vi "0_Camera_Acquisition_and_Image_Saving.vi"() -> ()   [LabVIEW 2020]
doc: "Overview: This example demonstrates usage of Deep Learning Toolkit for object detection based on pretrained network called YOLO https://pjreddie.com/darknet/yolo/\nToolkit's API is utilized to automatically create network architecture based network topology configuration file and load and initialize network's weights from weight file.\nRequirements: \n1. Deep Learning Toolkit for LabVIEW\n2. NI Vision Development Module"
uses:
  subVIs/Camera/Controls/Camera_Settings.ctl
  <vilib>/vision/driver/IMAQdx.llb/IMAQdx Camera Control Mode.ctl
  <vilib>/vision/driver/NI_Vision_Acquisition_Software.lvlib
panel:
  in  "Start Index":i32
  out "Loop Time":cluster{sgl, dbl}(graph)={0.28, 0.11247559999998202}
  out "Expected Time":sgl=0.28
  in  "Table Rot. Period":sgl=5.0
  in  "Label":string="good"
  in  "Camera_Settings":T1={"Camera_Resolution"=76, "Focus"=0, "Exposure"=2, "Gain"=13, "WhiteB."=5000} {"WhiteB." min=2800 max=6500 step=1; "Gain" max=255 step=1; "Exposure" min=0 max=6 step=1; "Focus" step=17}
  in  "# Imgs to Save":i32=25
  out "Count":i32=25
  in  "Start Saving?":bool
  out "Original_Image":T2(plugin-control)
  out "Processed_Image":T2(plugin-control)
  in  "Center Crop Size":i32=900
  in  "Dest. Folder":path=path "D:/Dataset_test"
  out "Loop Time (s)":dbl=0.11247559999998202
  in  "Stop":bool
  in  "Camera":refnum<k21>="cam1" caption="IMAQdx Session"
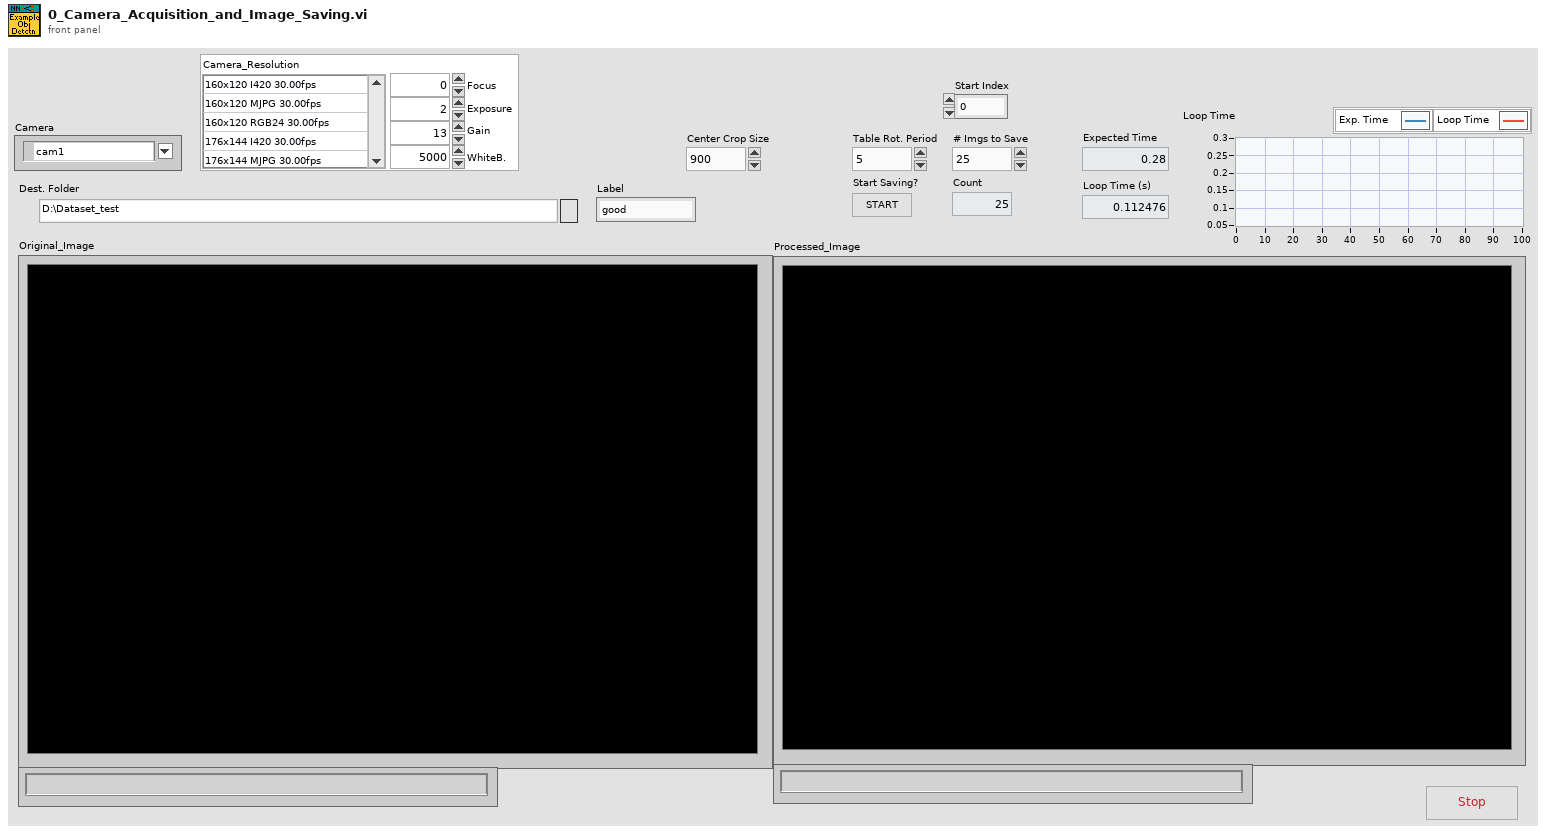
[diagram p1: front panel]
types:
  T1 = typedef "Camera_Settings.ctl" = cluster{"Camera_Resolution":i32, "Focus":u8, "Exposure":i32, "Gain":u32, "WhiteB.":i32}
  T2 = typedef "IMAQ Image.ctl" = refnum<image>
  T3 = typedef "NI_Vision_Acquisition_Software.lvlib/IMAQdx Camera Control Mode.ctl" = enum32{"Controller", "Listener"}
  T4 = typedef "Image Type" = u32
  T5 = typedef "IMAQdx.ctl" = refnum<k21>
  T6 = typedef "imagedata.ctl" = cluster{"image type":i32, "image depth":i32, "image":u8[], "mask":u8[], "colors":u32[], "Rectangle":cluster{"left":i16, "top":i16, "right":i16, "bottom":i16}}
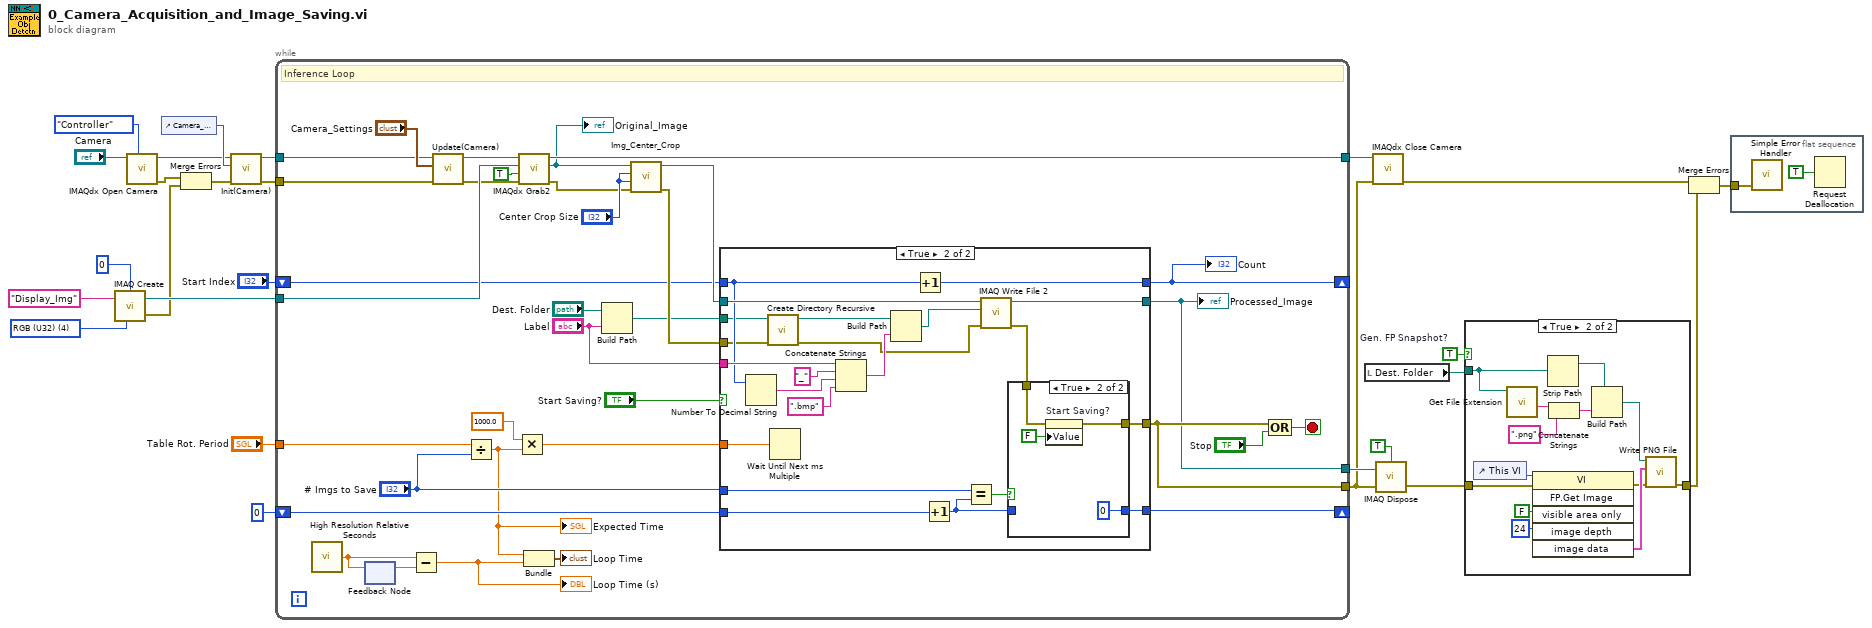
[diagram p0: block diagram]
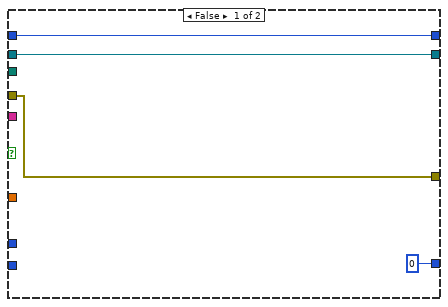
[diagram p2: hidden frame]
diagram:
  w4 = TRUE  # Gen. FP Snapshot?
  w18 = T4 4 items=["Grayscale (U8)", "Grayscale (I16)", "Grayscale (SGL)", "Complex (CSG)", "RGB (U32)", "HSL (U32)", "RGB (U64)", "Grayscale (U16)"] ("Image Type")
  n1 = call "IMAQ Create"("Border Size"=0, "Image Name"="Display_Img", "Image Type"=w18) -> ("New Image"=w24:T2, "error out"=w8:errorcluster)  [unwired: 2 in]
  n2 = call <vilib>:"IMAQdx Open Camera.vi"("Camera Control Mode"=IMAQdx_Camera_Control_Mode."Controller", "Session In"="Camera") -> ("error out"=w9:errorcluster, "Session Out"=w10:T5)  [unwired: 1 in, 7 out]
  n3 = control-ref of="Camera_Settings"() -> (w11:refnum<vi>)
  n4 = Merge Errors(w9, w8) -> (w12:errorcluster)
  n5 = call "Init(Camera).vi"("error in (no error)"=w12, "Camera_Settings_Ref"=w11, "Session in"=w10) -> ("error out"=w6:errorcluster, "Session out"=w7:T5)  [unwired: 7 in]
  n6 = while {
    tunnel: [w43] -> w25
    tunnel: w24 -> [w55]
    tunnel: [w57] -> w20
    tunnel: [w49] -> w14
    shift-right: [w48] -> _
    shift-left: "Start Index" -> [w47]
    tunnel: "Table Rot. Period" -> [w45]
    tunnel: w7 -> [w40]
    tunnel: w6 -> [w39]
    shift-right: [w31] -> _
    shift-left: 0 ("Camera Resolution") -> [w32]
    stop <- w58 stop-if-true
    # "Inference Loop"
    n7 = call <vilib>:"High Resolution Relative Seconds.vi"() -> ("relative seconds"=w59:dbl)
    n8 = feedback #1() -> (w60:dbl)  [unwired: 1 in]
    n9 = feedback-in #1(w59) -> ()
    n10 = Subtract(x=w59, y=w60) -> (x-y=w30:dbl)
    "Loop Time (s)" <- w30
    n11 = call "Update(Camera).vi"("error in (no error)"=w39, "Camera_Settings"="Camera_Settings", "Session in"=w40) -> ("error out"=w37:errorcluster, "Session out"=w38:T5)  [unwired: 7 in]
    n12 = Divide(x=w45, y="# Imgs to Save") -> (x/y=w27:sgl)
    "Expected Time" <- w27
    n13 = Multiply(x=sgl 1000.0, y=w27) -> (x*y=w28:sgl)
    n14 = call <vilib>:"IMAQdx Grab2.vi"("error in"=w37, "Wait for Next Buffer? (Yes)"=TRUE, "Image In"=w55, "Session In"=w38) -> ("error out"=w36:errorcluster, "Image Out"=w53:T2, "Session Out"=w57:T5)  [unwired: 4 in, 1 out]
    "Original_Image" <- w53
    n15 = Bundle(w27, w30) -> (→"Loop Time":cluster{sgl, dbl})  [unwired: 1 in]
    n16 = Build Path(base path="Dest. Folder", name or relative path="Label") -> (appended path=w34:path)
    n17 = call "Img_Center_Crop.vi"("error in (no error)"=w36, "height"="Center Crop Size", "width"="Center Crop Size", "Image In"=w53) -> ("error out"=w51:errorcluster, "Image Out"=w54:T2)  [unwired: 6 in]
    n18 = case shown="True" "Start Saving?" {
      tunnel: [w63 w75] -> w49
      tunnel: w34 -> [_ w68]
      tunnel: w54 -> [w64 w86]
      tunnel: [w64 w85] -> w43
      tunnel: w51 -> [w63 w66]
      tunnel: [w62 w73] -> w48
      tunnel: w47 -> [w62 w81]
      tunnel: "# Imgs to Save" -> [_ w84]
      tunnel: w28 -> [_ w83]
      tunnel: "Label" -> [_ w82]
      tunnel: w32 -> [_ w72]
      tunnel: [0 ("Camera Resolution") w71] -> w31
      frame False {
      }
      frame True {
        n19 = Number To Decimal String(number=w81) -> (decimal integer string=w80:string)  [unwired: 1 in]
        n20 = call <vilib>:"Create Directory Recursive.vi"("error in (no error)"=w66, "directory"=w68) -> ("error out"=w65:errorcluster, "directory copy"=w67:path)  [unwired: 3 in, 1 out]
        n21 = Wait Until Next ms Multiple(millisecond multiple=w83) -> ()  [unwired: 1 out]
        n22 = Concatenate Strings(w82, "_" ("string"), w80, ".bmp") -> (w78:string)
        n23 = Build Path(base path=w67, name or relative path=w78) -> (appended path=w69:path)
        n24 = Increment(x=w81) -> (x+1=w73:i32)
        n25 = Increment(x=w72) -> (x+1=w70:i32)
        n26 = Equal?(x=w84, y=w70) -> (x = y?=w77:bool)
        n27 = call-poly "IMAQ Write File 2"("error in (no error)"=w65, "File Path"=w69, "Image"=w86) -> ("error out"=w76:errorcluster, "Image Out (duplicate)"=w85:T2)  [unwired: 7 in]
        n28 = case shown="True" w77 {
          tunnel: w76 -> [w88 w91]
          tunnel: [w88 w90] -> w75
          tunnel: w70 -> [w87 _]
          tunnel: [w87 0 ("Camera Resolution")] -> w71
          frame False {
          }
          frame True {
            n29 = property on="Start Saving?" class="Bool (strict)"(error in=w91, "Value"=FALSE ("Start Saving?")) -> (error out=w90:errorcluster)  [unwired: 1 in, 1 out]
          }
        }
      }
    }
    "Processed_Image" <- w43
    "Count" <- w48
    n30 = Compound Arithmetic op=OR(w49, "Stop") -> (w58:bool)
  }
  n31 = local read "Dest. Folder"() -> (w1:path)
  n32 = call <vilib>:"IMAQdx Close Camera.vi"("error in"=w14, "Session In"=w20) -> ("error out"=w19:errorcluster)  [unwired: 9 out]
  n33 = call "IMAQ Dispose"("All Images? (No)"=TRUE, "Image"=w25, "error in (no error)"=w14) -> ("error out"=w3:errorcluster)  [unwired: 3 in]
  n34 = case shown="True" w4 {
    tunnel: w3 -> [w93 w96]
    tunnel: [w93 w95] -> w2
    tunnel: w1 -> [_ w94]
    frame False {
    }
    frame True {
      n35 = control-ref of="This VI"() -> (w106:refnum<vi>)
      n36 = call <vilib>:"Get File Extension.vi"("file"=w94) -> ("filename without extension"=w101:string)  [unwired: 6 in, 4 out]
      n37 = invoke class="VI" method="FP.Get Image"(reference=w106, error in=w96, "visible area only"=FALSE ("Visible Area Only"), "image depth"=24 ("Image Depth")) -> (error out=w102:errorcluster, "image data"=w103:T6)  [unwired: 2 in, 4 out]
      n38 = Strip Path(path=w94) -> (stripped path=w98:path)  [unwired: 1 out]
      n39 = Concatenate Strings(w101, ".png" ("string")) -> (w99:string)
      n40 = Build Path(base path=w98, name or relative path=w99) -> (appended path=w97:path)
      n41 = call <vilib>:"Write PNG File.vi"("error in (no error)"=w102, "image data"=w103, "path to PNG file"=w97) -> ("error out"=w95:errorcluster)  [unwired: 7 in, 1 out]
    }
  }
  n42 = Merge Errors(w19, w2) -> (w23:errorcluster)
  n43 = flat-sequence {
    tunnel: w23 -> [w107]
    frame #0 {
      n44 = call <vilib>:"Simple Error Handler.vi"("error in (no error)"=w107) -> ()  [unwired: 4 in, 5 out]
      n45 = Request Deallocation(TRUE ("flag")) -> ()
    }
  }
